vi "Arm Globals.vi"() -> ()   [LabVIEW 2013]
uses:
  ROS/RosMessages/Clusters/JointCommand.ctl
  <vilib>/Analysis/Matrix/Datatypes/RealMatrix.ctl
  <vilib>/Analysis/Matrix/NI_Matrix.lvlib
panel:
  in  "L:Joints":dbl[](array[numeric])=[-0.416, -0.52, 1.12, -3.856, -0.084, -0.176, 0.14]
  in  "R:Joints":dbl[](array[numeric])=[-0.416, -0.52, 1.12, -3.856, -0.084, -0.176, 0.14]
  in  "R: Right of Post":dbl[](array[numeric])=[-1.0, -80.0, 0.0, 120.0, 0.0, 50.0, 0.0] format="%.3f"
  in  "L: Left of Post":dbl[](array[numeric])=[0.0, -80.0, 0.0, 150.0, 0.0, 20.0, 0.0] format="%.3f"
  in  "L: Joint Locations":cluster{"Name":string, "Joints":dbl[]}[](array[cluster])
  in  "L:Matrix Locations":T2(array[cluster])=[{"Label"="Tray", "Joints"=[-84.57275380961154, -47.61474603934222, -7.866210928511545, 84.11132802888879, 6.416015617668634, 53.811035094761934, -9.426269520478916], "T"=[[-0.5988876569529115, 0.800833050235473, 0.0, -366.00520548648257], [-0.800833050235473, -0.5988876569529115, 0.0, -711.8913976413369], [0.0, 0.0, 1.0, -363.72215324721117], [0.0, 0.0, 0.0, 1.0]]}] {"T" format="%#.3g"}
  in  "R: Joint Locations":cluster{"Name":string, "Joints":dbl[]}[](array[cluster])
  in  "L: Right of Post":dbl[](array[numeric])=[-25.0, -80.0, 0.0, 150.0, 0.0, 20.0, 0.0] format="%.3f"
  in  "L:tTg":T1=[[-1.0, 0.0, 0.0, 0.0], [0.0, 1.0, 0.0, 0.0], [0.0, 0.0, -1.0, 99.0], [0.0, 0.0, 0.0, 1.0]]
  in  "L: Interpolated  Locations":T3(array[cluster])=[{"Label"="Table", "Joints"=[44.89013666745554, -43.242187450588595, -0.1098632811244629, 63.3471678963653, 0.1318359373493555, 69.71923820158416, -0.021972656224892577], "Far Left"={"Absolute"=[175.0, 1025.0], "Robot"=[633.4344811440129, -146.22877470140702, -111.02594930708905, -4.693050489224001]}, "Far Right"={"Absolute"=[175.0, 1025.0], "Robot"=[633.4344811440129, -146.22877470140702, -111.02594930708905, -4.693050489224001]}, "Near Left"={"Absolute"=[175.0, 1025.0], "Robot"=[633.4344811440129, -146.22877470140702, -111.02594930708905, -4.693050489224001]}, "Near Right"={"Absolute"=[175.0, 1025.0], "Robot"=[633.4344811440129, -146.22877470140702, -111.02594930708905, -4.693050489224001]}}, {"Label"="Mat", "Joints"=[44.23095698070876, -63.984374926887185, 5.822753899596534, 95.62499989073251, -2.9443359341356055, 58.60107415178852, 6.965332023290947], "Far Left"={"Absolute"=[250.0, 545.0, 0.0, 0.0], "Robot"=[672.1715994990807, 48.007748317552725, -89.34911586830711, -0.8655128374424802]}, "Far Right"={"Absolute"=[250.0, 25.0, 0.0, 0.0], "Robot"=[665.1874122546096, -469.0278466112149, -103.34889570552687, -1.1608424316603774]}, "Near Left"={"Absolute"=[25.0, 545.0, 0.0, 0.0], "Robot"=[441.4908301445158, 48.901036437406674, -90.12517532297716, 0.03683219744794118]}, "Near Right"={"Absolute"=[25.0, 25.0, 0.0, 0.0], "Robot"=[437.9607504937842, -467.7872050538727, -109.66068983948531, -0.8484520588115468]}}] {"Joints" format="%.2f"}
  in  "R: Left of Post":dbl[](array[numeric])=[1.0, -80.0, 0.0, 120.0, 0.0, 50.0, 0.0] format="%.3f"
  in  "R: Interpolated  Locations":T3(array[cluster])=[{"Label"="Table", "Joints"=[44.89013666745554, -43.242187450588595, -0.1098632811244629, 63.3471678963653, 0.1318359373493555, 69.71923820158416, -0.021972656224892577], "Far Left"={"Absolute"=[175.0, 1025.0], "Robot"=[633.4344811440129, -146.22877470140702, -111.02594930708905, -4.693050489224001]}, "Far Right"={"Absolute"=[175.0, 1025.0], "Robot"=[633.4344811440129, -146.22877470140702, -111.02594930708905, -4.693050489224001]}, "Near Left"={"Absolute"=[175.0, 1025.0], "Robot"=[633.4344811440129, -146.22877470140702, -111.02594930708905, -4.693050489224001]}, "Near Right"={"Absolute"=[175.0, 1025.0], "Robot"=[633.4344811440129, -146.22877470140702, -111.02594930708905, -4.693050489224001]}}, {"Label"="Mat", "Joints"=[44.23095698070876, -63.984374926887185, 5.822753899596534, 95.62499989073251, -2.9443359341356055, 58.60107415178852, 6.965332023290947], "Far Left"={"Absolute"=[250.0, 545.0, 0.0, 0.0], "Robot"=[672.1715994990807, 48.007748317552725, -89.34911586830711, -0.8655128374424802]}, "Far Right"={"Absolute"=[250.0, 25.0, 0.0, 0.0], "Robot"=[665.1874122546096, -469.0278466112149, -103.34889570552687, -1.1608424316603774]}, "Near Left"={"Absolute"=[25.0, 545.0, 0.0, 0.0], "Robot"=[441.4908301445158, 48.901036437406674, -90.12517532297716, 0.03683219744794118]}, "Near Right"={"Absolute"=[25.0, 25.0, 0.0, 0.0], "Robot"=[437.9607504937842, -467.7872050538727, -109.66068983948531, -0.8484520588115468]}}] {"Joints" format="%.2f"}
  in  "Configuration Path":path=path "C:/Program Files/Labview/user.lib/ROSforLV_0.1/Devices/Baxter/Cartesian/Object Locations.ini"
  in  "R:Effort":dbl[](array[numeric])=[-0.416, -0.52, 1.12, -3.856, -0.084, -0.176, 0.14]
  in  "R:Matrix Locations":T2(array[cluster])=[{"Label"="Tray", "Joints"=[-84.57275380961154, -47.61474603934222, -7.866210928511545, 84.11132802888879, 6.416015617668634, 53.811035094761934, -9.426269520478916], "T"=[[-0.5988876569529115, 0.800833050235473, 0.0, -366.00520548648257], [-0.800833050235473, -0.5988876569529115, 0.0, -711.8913976413369], [0.0, 0.0, 1.0, -363.72215324721117], [0.0, 0.0, 0.0, 1.0]]}] {"T" format="%#.3g"}
  in  "R:tTc":T1=[[-1.0, 0.0, 0.0, 40.0], [0.0, 1.0, 0.0, 12.0], [0.0, 0.0, -1.0, 0.0], [0.0, 0.0, 0.0, 1.0]]
  in  "R:tTg":T1=[[-1.0, 0.0, 0.0, 0.0], [0.0, 1.0, 0.0, 0.0], [0.0, 0.0, -1.0, 99.0], [0.0, 0.0, 0.0, 1.0]]
  in  "L:Command":T4={"Mode"=enum."Position", "Arm Angles"=[], "Angle Names"=["right_s0", "left_s1", "left_e0", "left_e1", "left_w0", "left_w1", "left_w2"]}
  in  "Stop":bool
  out "L:Status":string="Home"
  in  "L:Jt Limits":dbl[][](array[numeric])=[[141.0, -51.0], [60.0, -123.0], [173.5, -173.5], [150.0, -3.0], [175.25, -175.25], [120.0, -90.0], [175.25, -175.25]] format="%.2f"
  in  "L:End":i32
  in  "L:Pause":bool
  in  "R:Command":T4={"Mode"=enum."Position", "Arm Angles"=[0.7792622393554688, -0.08360195284423828, -0.001917475982666016, 1.5109710743408205, -0.001917475982666016, 0.2592427528564453, -0.001917475982666016], "Angle Names"=["left_s0", "left_s1", "left_e0", "left_e1", "left_w0", "left_w1", "left_w2"]}
  out "R:Status":string="Initial"
  in  "R:Jt Limits":dbl[][](array[numeric])=[[51.0, -141.0], [60.0, -123.0], [173.5, -173.5], [150.0, -3.0], [175.25, -175.25], [120.0, -90.0], [175.25, -175.25]] format="%.2f"
  in  "R:End":i32
  in  "R:Pause":bool
  # "Tool plate to gripper fingers"
  # "Tool Plate to camera"
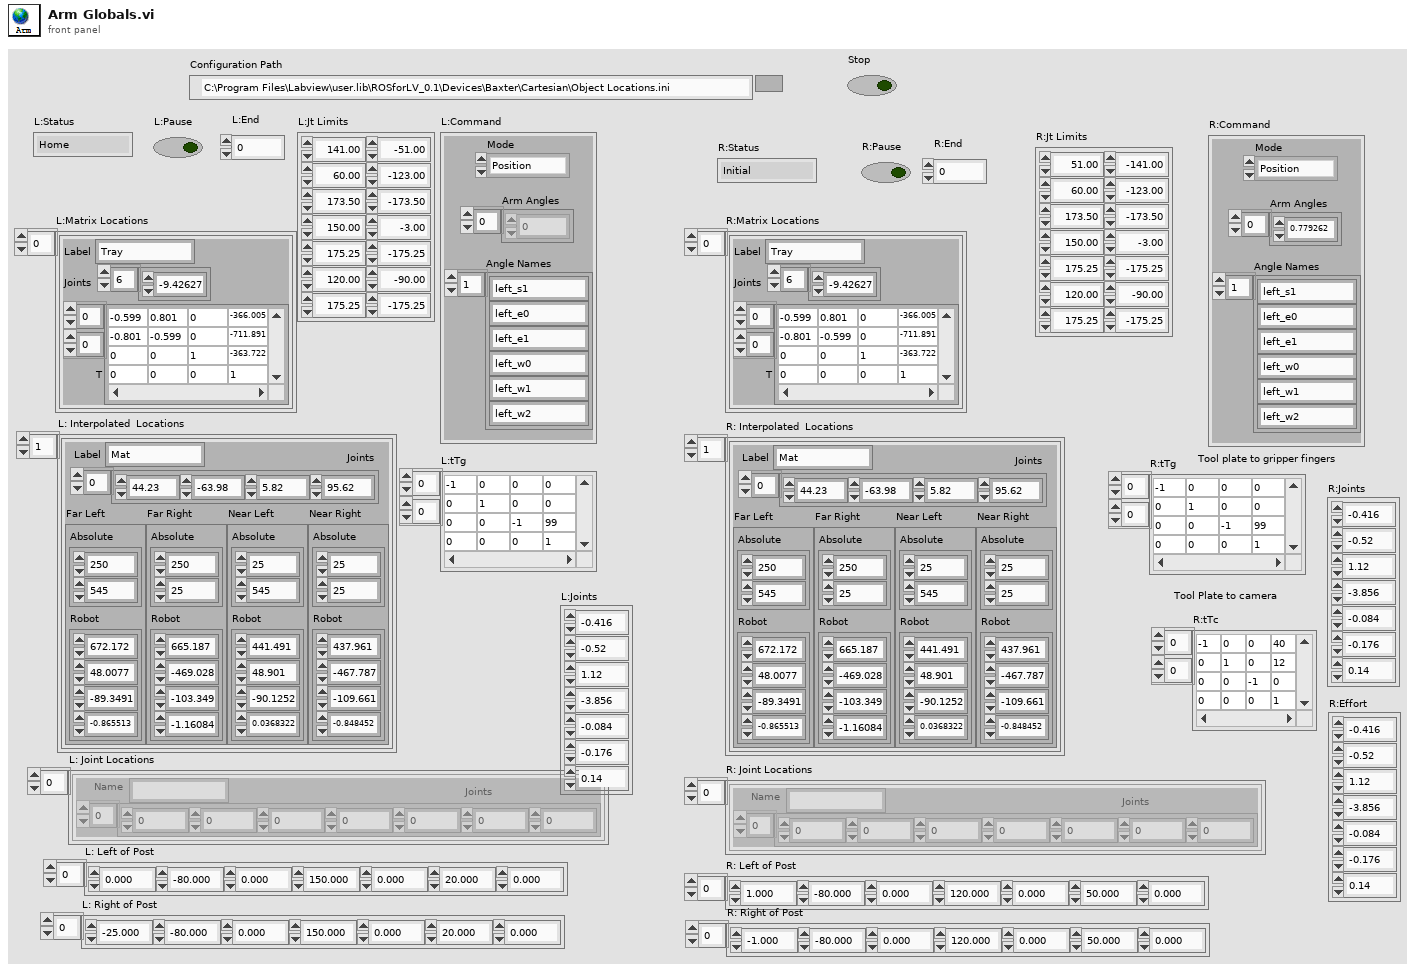
[diagram p1: front panel]
types:
  T1 = typedef "NI_Matrix.lvlib/RealMatrix.ctl" = dbl[][]
  T2 = cluster{"Label":string, "Joints":dbl[], "T":T1}[]
  T3 = cluster{"Label":string, "Joints":dbl[], "Far Left":cluster{"Absolute":dbl[], "Robot":dbl[]}, "Far Right":cluster{"Absolute":dbl[], "Robot":dbl[]}, "Near Left":cluster{"Absolute":dbl[], "Robot":dbl[]}, "Near Right":cluster{"Absolute":dbl[], "Robot":dbl[]}}[]
  T4 = typedef "JointCommand.ctl" = cluster{"Mode":enum32{"", "Position", "Velocity", "Effort"}, "Arm Angles":dbl[], "Angle Names":string[]}
diagram:
